vi "Initialisierung.vi"() -> ()   [LabVIEW 2010]
uses:
  <vilib>/Utility/error.llb/DialogType.ctl
panel:
  out "Initialisierung":bool
  out "Versuch Nr.":i32
  out "message":string=" ANWEISUNGEN:\r\rAllgemeine Nutzung:  Bei der Benutzung von SubVIs, die die Fehler(Eingang)-/Fehler(Ausgang)- (oder Fehler-I/O-) Struktur verwenden, platzieren Sie diesen Handler dort, wo Sie den Benutzer auf aufgetretene Fehler hinweisen wollen, in der Regel am Ende eines I/O-Datenpfads als letzte Aktion des Programms.  Wenn der Fehlerstatus einen Fehler angibt, erzeugt der Handler eine Nachricht, die den Fehler und dessen Ursprung beschreibt.  Ist Dialogtyp = 1 (Voreinstellung), wird die Fehlermeldung angezeigt und der Benutzer kann diese bestätigen.  Ist Dialogtyp = 2, kann der Benutzer die Meldung bestätigen oder die Programm-Ausführung abbrechen. Der Abbruch eines Programms mit aktiver I/O wird jedoch nicht empfohlen.  Ist der Dialogtyp = 0, wird keine Meldung angezeigt; dieser Modus wird verwendet, um Fehler programmatisch zu behandeln, aus diesem Grunde sind auch die Fehlerausgangs-Cluster mit individuellen Terminals verbunden.  \r\rAndere Nutzungsmöglichkeit:\n\r\nLokales Testen.  Um einen Fehlercode eines SubVI oder einer Funktion zu testen, die keine Fehler-I/O-Struktur beinhalten, kann deren Fehlercode und ein Quellen-String mit den lokalen Fehlercode- und Quellenstring-Eingängen verbunden werden.  Wenn der Fehlerstatus keinen Fehler anzeigt und der Fehlercode ungleich 0 ist, werden der lokale Code und der String des Fehlereingangs-Werts ersetzt und Fehler? wird auf TRUE (FEHLER) gesetzt." caption="Nachricht"
  out "source out":string caption="Quelle (Ausgang)"
  out "code out":i32 caption="Code (Ausgang)" format="%0.0f"
  in  "Operation (0:Öffnen)":T1(ring)
  in  "Dateipfad (Dialog verwenden)":path
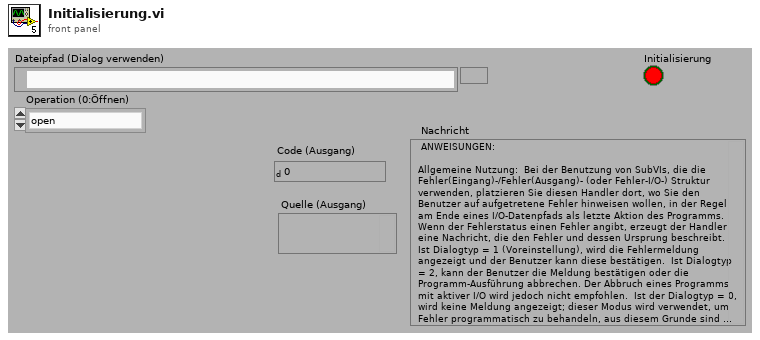
[diagram p1: front panel]
types:
  T1 = enum16{"open", "replace", "create", "open or create", "replace or create", "replace or create with confirmation"}
  T2 = typedef "DialogType.ctl" = u16
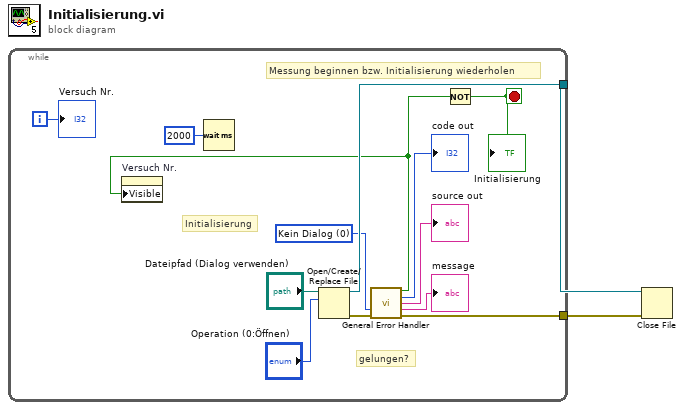
[diagram p0: block diagram]
diagram:
  n1 = while {
    tunnel: [w13] -> w2
    tunnel: [w6] -> w1
    i -> [w5]
    stop <- w11 stop-if-true
    w10 = T2 0 items=["Kein Dialog", "OK-Meldung", "Dialog zum Fortsetzen oder Anhalten", "OK-Meldung + Warnungen", "Weiter/Stopp + Warnung"] ("type of dialog (OK msg:1)")
    # "Messung beginnen bzw. Initialisierung wiederholen"
    # "gelungen?"
    # "Initialisierung"
    n2 = Wait (ms)(milliseconds to wait=u32 2000 ("Zu wartende ms")) -> ()  [unwired: 1 out]
    n3 = Open/Create/Replace File(file path (use dialog)="Dateipfad (Dialog verwenden)", operation (0:open)="Operation (0:Öffnen)") -> (refnum out=w13:refnum<file>, error out=w12:errorcluster)  [unwired: 4 in, 1 out]
    n4 = call <vilib>:"General Error Handler.vi"("type of dialog (OK msg:1)"=w10, "error in (no error)"=w12) -> ("error?"=w3:bool, "code out"=→"code out":i32, "source out"=→"source out":string, "message"=→"message":string, "error out"=w6:errorcluster)  [unwired: 9 in]
    n5 = property on="Versuch Nr." class="DigNum (strict)"("Visible"=w3) -> ()  [unwired: 2 in, 2 out]
    n6 = Not(x=w3) -> (.not. x?=w11:bool)
    "Initialisierung" <- w11
    "Versuch Nr." <- w5
  }
  n7 = Close File(refnum=w2, error in=w1) -> ()  [unwired: 2 out]
